vi "DB Import Action - Create Chans.vi"(8 "error in (no error)":errorcluster, 10 "selected path":path, 11 "Node Ptr":u64) -> (0 "error out":errorcluster, 2 "selected path out":path caption="selected path", 3 "Node Ptr dup":u64, 5 "Item Ref":T1 format="%.0x")   [LabVIEW 2013, in "AIT 664 Custom Device.lvlib"]
doc: "Load xml file and populate Veristand with configuration"
uses:
  AIT 664 Custom Device.lvlib
  <vilib>/NI Veristand/Custom Device API/Custom Device Item Ref.ctl
  <vilib>/NI Veristand/Custom Device API/Custom Device API.lvlib
panel:
  # "Loading Simulyzer Configuration...\nPlease Wait"
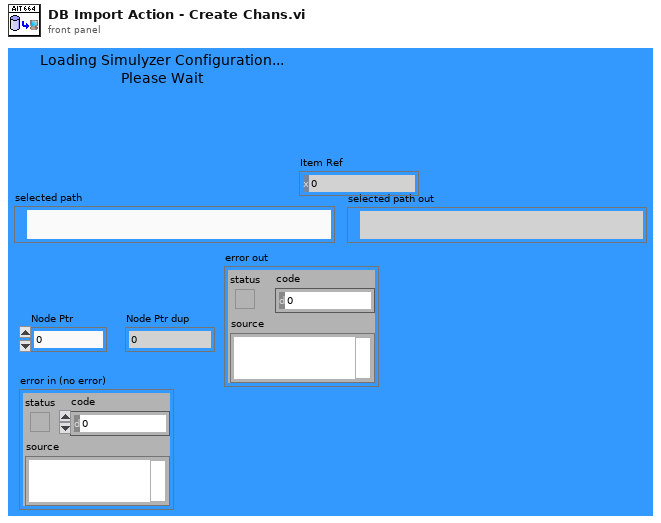
[diagram p1: front panel]
types:
  T1 = typedef "Custom Device API.lvlib/Custom Device Item Ref.ctl" = u64
  T2 = typedef "AIT 664 Custom Device.lvlib/664 - XML Device Description.ctl" = cluster{"Name":string, "Network Speed":string, "MAC Address":string, "VISA Resource Name":string, "End Systems":T3[]}
  T3 = typedef "AIT 664 Custom Device.lvlib/664 - XML End System Description.ctl" = cluster{"Name":string, "Id":u32, "MAC Address":string, "Output VLs":T4[], "Input VLs":T8[]}
  T4 = typedef "AIT 664 Custom Device.lvlib/664 - XML Output VL.ctl" = cluster{"Name":string, "VL Id":u32, "Tx Message Ports":T5[]}
  T5 = typedef "AIT 664 Custom Device.lvlib/664 - XML Tx Message Port.ctl" = cluster{"Name":string, "Port Id":u32, "Sampling Type":T6, "Parameters":T7[], "Source IP Address":string, "Source UDP Port":u32, "Destination IP Address":string, "Destination UDP Port":u32, "Tx Rate (ms)":u32}
  T6 = typedef "AIT 664 Custom Device.lvlib/664 - Sampling Type.ctl" = enum16{"Com Udp", "Com Udp Queuing", "Sap Udp", "Sap Ip", "Sap Mac", "Unknown"}
  T7 = typedef "AIT 664 Custom Device.lvlib/664 -Param.ctl" = cluster{"name":string, "firstByte":i32, "startBit":i32, "numberBits":i32, "scaleFactor":dbl, "scaleOffset":dbl, "signed":bool}
  T8 = typedef "AIT 664 Custom Device.lvlib/664 - XML Input VL.ctl" = cluster{"Name":string, "VL Id":u32, "Rx Message Ports":T9[]}
  T9 = typedef "AIT 664 Custom Device.lvlib/664 - XML Rx Message Port.ctl" = cluster{"Name":string, "Port Id":u32, "Sampling Type":T6, "Parameters":T7[], "Source IP Address":string, "Source UDP Port":u32, "Destination IP Address":string, "Destination UDP Port":u32, "Rx Rate (ms)":u32, "Buffer Depth":u32}
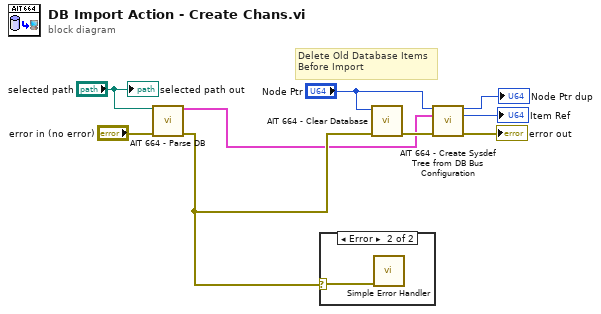
[diagram p0: block diagram]
diagram:
  # "Delete Old Database Items\nBefore Import"
  n1 = call "AIT 664 - Parse DB.vi"("Path in"="selected path", "error in (no error)"="error in (no error)") -> ("664 Device"=w1:T2, "error out"=w2:errorcluster)  [unwired: 12 in]
  n2 = case shown="Error" w2 {
    selector: w2 -> [_ w10]
    frame No Error {
    }
    frame Error {
      n3 = call <vilib>:"Simple Error Handler.vi"("error in (no error)"=w10) -> ()  [unwired: 4 in, 5 out]
    }
  }
  n4 = call "AIT 664 - Clear Database.vi"("error in (no error)"=w2, "Node Ptr"="Node Ptr") -> ("error out"=w4:errorcluster)  [unwired: 9 in]
  n5 = call "AIT 664 - Create Sysdef Tree from DB Bus Configuration.vi"("Section Ref in"="Node Ptr", "664 Device"=w1, "error in"=w4) -> ("Section Ref out"=→"Node Ptr dup":T1, "Item Ref"=→"Item Ref":T1, "error out"=→"error out":errorcluster)  [unwired: 10 in]
  "selected path out" <- "selected path"
